vi "GetSwitchPos.vi"(4 "error in (no error)":errorcluster, 7 "Circuit ID":i32=7201 format="%_4g") -> (0 "Error out":errorcluster, 1 "Paired = 1":i32, 2 "Switch Position Verify  Sense":string, 3 "Position (0=open, 1=closed)":i32)   [LabVIEW 2009]
doc: "Reads a value from the 34980. \nAssumes that you have scanned the 34980 to store the values."
panel:
  out "Pulsed = 1":i32
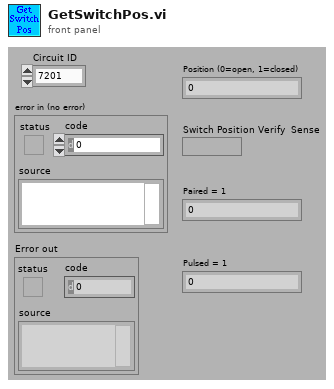
[diagram p1: front panel]
types:
  T1 = enum16{"N1911A", "Siggen", "34980a", "E4418B", "Rvp8"}
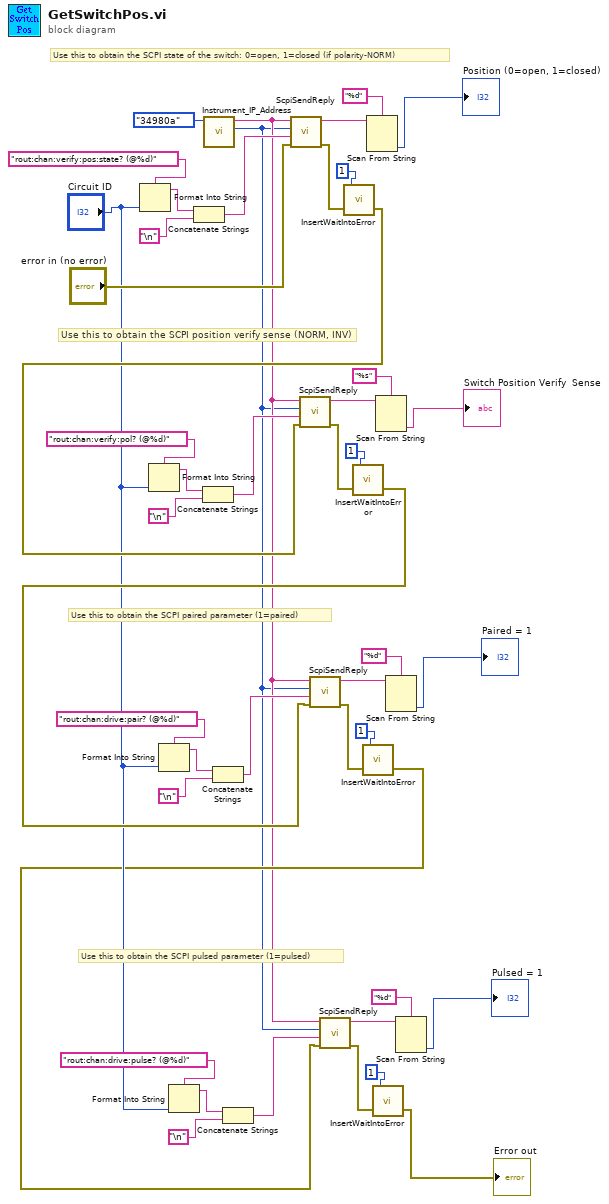
[diagram p0: block diagram]
diagram:
  # "Use this to obtain the SCPI pulsed parameter (1=pulsed)"
  # "Use this to obtain the SCPI paired parameter (1=paired)"
  # "Use this to obtain the SCPI position verify sense (NORM, INV)"
  # "Use this to obtain the SCPI state of the switch: 0=open, 1=closed (if polarity-NORM)"
  n1 = Format Into String(format string="rout:chan:verify:pos:state? (@%d)", "Circuit ID") -> (resulting string=w40:string)  [unwired: 2 in, 1 out]
  n2 = Format Into String(format string="rout:chan:verify:pol? (@%d)", "Circuit ID") -> (resulting string=w32:string)  [unwired: 2 in, 1 out]
  n3 = Format Into String(format string="rout:chan:drive:pair? (@%d)", "Circuit ID") -> (resulting string=w23:string)  [unwired: 2 in, 1 out]
  n4 = Format Into String(format string="rout:chan:drive:pulse? (@%d)", "Circuit ID") -> (resulting string=w11:string)  [unwired: 2 in, 1 out]
  n5 = Concatenate Strings(w40, "\n") -> (w38:string)
  n6 = Concatenate Strings(w32, "\n") -> (w30:string)
  n7 = call "Instrument_IP_Address.vi"("Instrument"=T1."34980a") -> ("Port"=w1:u16, "IP Address"=w2:string)  [unwired: 9 in]
  n8 = Concatenate Strings(w23, "\n") -> (w21:string)
  n9 = Concatenate Strings(w11, "\n") -> (w9:string)
  n10 = call "ScpiSendReply.vi"("error in (no error)"="error in (no error)", "Command"=w38, "TCP port"=w1, "IP Address"=w2) -> ("Error out"=w37:errorcluster, "Reply"=w44:string)  [unwired: 5 in]
  n11 = call "InsertWaitIntoError.vi"("error in (no error)"=w37, "Wait (msecs)"=1) -> ("error out"=w18:errorcluster)  [unwired: 1 in]
  n12 = call "ScpiSendReply.vi"("error in (no error)"=w18, "Command"=w30, "TCP port"=w1, "IP Address"=w2) -> ("Error out"=w29:errorcluster, "Reply"=w34:string)  [unwired: 5 in]
  n13 = call "InsertWaitIntoError.vi"("error in (no error)"=w29, "Wait (msecs)"=1) -> ("error out"=w17:errorcluster)  [unwired: 1 in]
  n14 = call "ScpiSendReply.vi"("error in (no error)"=w17, "Command"=w21, "TCP port"=w1, "IP Address"=w2) -> ("Error out"=w20:errorcluster, "Reply"=w26:string)  [unwired: 5 in]
  n15 = call "InsertWaitIntoError.vi"("error in (no error)"=w20, "Wait (msecs)"=1) -> ("error out"=w4:errorcluster)  [unwired: 1 in]
  n16 = call "ScpiSendReply.vi"("error in (no error)"=w4, "Command"=w9, "TCP port"=w1, "IP Address"=w2) -> ("Error out"=w8:errorcluster, "Reply"=w14:string)  [unwired: 5 in]
  n17 = Scan From String(format string="%d", input string=w44) -> (output 1=→"Position (0=open, 1=closed)":i32)  [unwired: 3 in, 3 out]
  n18 = call "InsertWaitIntoError.vi"("error in (no error)"=w8, "Wait (msecs)"=1) -> ("error out"=→"Error out":errorcluster)  [unwired: 1 in]
  n19 = Scan From String(format string="%s", input string=w34) -> (output 1=→"Switch Position Verify  Sense":string)  [unwired: 3 in, 3 out]
  n20 = Scan From String(format string="%d", input string=w26) -> (output 1=→"Paired = 1":i32)  [unwired: 3 in, 3 out]
  n21 = Scan From String(format string="%d", input string=w14) -> (output 1=→"Pulsed = 1":i32)  [unwired: 3 in, 3 out]
